vi "Remove All.vi"(8 "error in (no error)":errorcluster, 11 "dsf refnum":T1) -> (0 "error out":errorcluster, 3 "dsf refnum out":T1)   [LabVIEW 2017, in "DSF Configuration.lvlib" / "Configuration Session.lvclass"]
doc: "Removes a section from the configuration data identified by <B>dsf refnum</B>."
uses:
  Configuration/Session/Configuration Session.lvclass
  Controls/DSF Config Data RefNum.ctl
  Private/Controls/DSF File Format/Internal.DSF Group with ID.ctl
  Private/Controls/DSF File Format/Internal.DSF Group Info.ctl
  Controls/DSF Timing Info.ctl
  Private/Controls/DSF File Format/Internal.DSF Transfer with ID.ctl
  Private/Controls/DSF File Format/Internal.DSF Transfer Info.ctl
  Private/Controls/DSF File Format/Internal.DSF Channel with ID.ctl
  Private/Controls/DSF File Format/Internal.DSF Channel Info.ctl
  Private/Controls/DSF File Format/Internal.DSF Settings with ID.ctl
  Private/Controls/DSF File Format/Internal.DSF Settings Info.ctl
  Private/Controls/DSF File Format/Internal.DSF Plugin with ID.ctl
  Private/Controls/DSF File Format/Internal.DSF Plugin Info.ctl
  DSF Configuration.lvlib
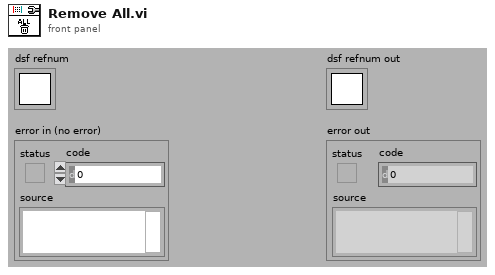
[diagram p1: front panel]
types:
  T1 = typedef "DSF Configuration.lvlib/DSF Config Data RefNum.ctl" = refnum<k1>
  T2 = typedef "DSF Configuration.lvlib/Configuration Session.lvclass/Internal.DSF Plugin with ID.ctl" = cluster{"id":string, "values":T3}
  T3 = typedef "DSF Configuration.lvlib/Configuration Session.lvclass/Internal.DSF Plugin Info.ctl" = cluster{"type":string, "timing":T4, "group ids":string[], "settings id":string}
  T4 = typedef "DSF Configuration.lvlib/DSF Timing Info.ctl" = cluster{"priority":u64, "decimation":u64, "offset":u64}
  T5 = typedef "DSF Configuration.lvlib/Configuration Session.lvclass/Internal.DSF Settings with ID.ctl" = cluster{"id":string, "values":T6}
  T6 = typedef "DSF Configuration.lvlib/Configuration Session.lvclass/Internal.DSF Settings Info.ctl" = cluster{"key":string, "value":string}[]
  T7 = typedef "DSF Configuration.lvlib/Configuration Session.lvclass/Internal.DSF Channel with ID.ctl" = cluster{"id":string, "values":T8}
  T8 = typedef "DSF Configuration.lvlib/Configuration Session.lvclass/Internal.DSF Channel Info.ctl" = cluster{"count":u64, "buffer offset":u64, "data type":i32, "settings id":string}
  T9 = typedef "DSF Configuration.lvlib/Configuration Session.lvclass/Internal.DSF Transfer with ID.ctl" = cluster{"id":string, "values":T10}
  T10 = typedef "DSF Configuration.lvlib/Configuration Session.lvclass/Internal.DSF Transfer Info.ctl" = cluster{"byte order":i32, "channel ids":string[], "settings id":string}
  T11 = typedef "DSF Configuration.lvlib/Configuration Session.lvclass/Internal.DSF Group with ID.ctl" = cluster{"id":string, "values":T12}
  T12 = typedef "DSF Configuration.lvlib/Configuration Session.lvclass/Internal.DSF Group Info.ctl" = cluster{"direction":i32, "timing":T4, "transfer ids":string[], "settings id":string}
  T13 = typedef "DSF Configuration.lvlib/Configuration Session.lvclass/DSF Configuration Reference.ctl" = refnum<data-value>
  T14 = typedef "DSF Configuration.lvlib/Configuration Session.lvclass/Internal.DSF Configuration.ctl" = cluster{"dsfversion":T15, "version":T15, "plugins":T2[], "groups":T11[], "transfers":T9[], "channels":T7[], "settings":T5[]}
  T15 = typedef "DSF Configuration.lvlib/DSF Version Info.ctl" = cluster{"major":u32, "minor":u32, "fix":u32, "build":string}
  T16 = cluster{"dsf configuration":T14, "path":path, "dirty":bool}
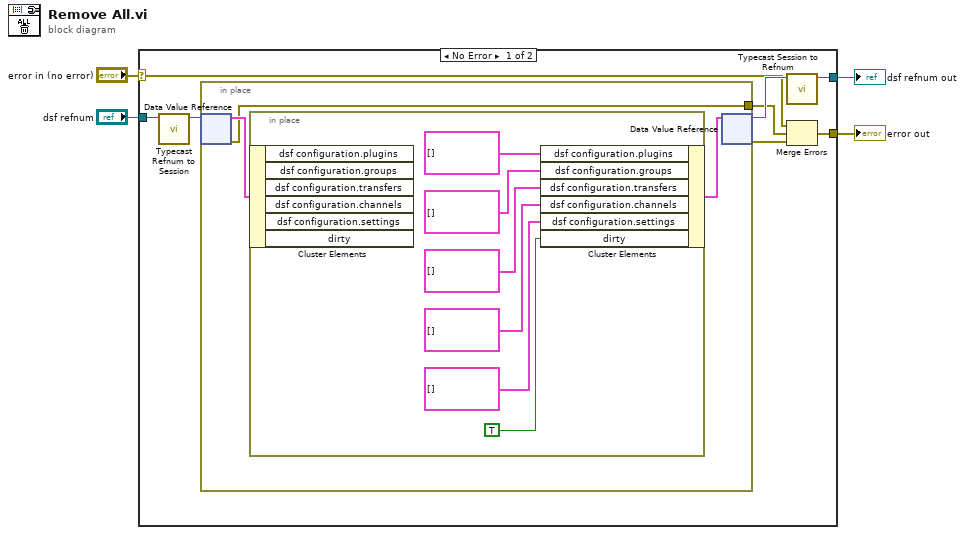
[diagram p0: block diagram]
diagram:
  n1 = case shown="No Error" "error in (no error)" {
    selector: "error in (no error)" -> [w8 w23]
    tunnel: [w5 w23] -> w1
    tunnel: [w11 w22] -> w2
    tunnel: "dsf refnum" -> [w12 w22]
    frame No Error {
      n2 = call "Typecast Refnum to Session.vi"("dsf refnum in"=w12) -> ("DSF Configuration Session out"=w10:T13)  [unwired: 10 out]
      n3 = in-place {
        in-place-border: [w13] -> w7
        n4 = in-place-dvr #1(w10) -> (w15:T16, w13:errorcluster)
        n5 = in-place {
          n6 = in-place-cluster #2(w15) -> ()  [unwired: 6 out]
          n7 = in-place-cluster #2("dsf configuration.plugins"=T2[] [], "dsf configuration.groups"=T11[] [], "dsf configuration.transfers"=T9[] [], "dsf configuration.channels"=T7[] [], "dsf configuration.settings"=T5[] [], "dirty"=TRUE) -> (w14:T16)
        }
        n8 = in-place-dvr #1(w14) -> (w9:T13, w6:errorcluster)
      }
      n9 = call "Typecast Session to Refnum.vi"("DSF Configuration Session in"=w9) -> ("dsf refnum out"=w11:T1)  [unwired: 10 out]
      n10 = Merge Errors(w8, w7, w6) -> (w5:errorcluster)
    }
    frame Error {
    }
  }
  "error out" <- w1
  "dsf refnum out" <- w2
